vi "RTM SLSC DisableEnable.vi"(11 "Node Ptr":T1=18446744073709551615 format="%.0x") -> ()   [LabVIEW 2015, in "SLSC-12201 DIO System Explorer.lvlib"]
uses:
  SLSC-12201 DIO System Explorer.lvlib
  <vilib>/NI Veristand/Custom Device API/Custom Device Item Ref.ctl
  Shared/Constants.vi
  <vilib>/NI Veristand/Custom Device API/Custom Device API.lvlib
  Shared/SLSC-12201 DIO Shared.lvlib
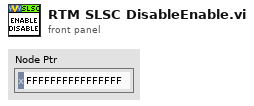
[diagram p1: front panel]
types:
  T1 = typedef "Custom Device API.lvlib/Custom Device Item Ref.ctl" = u64
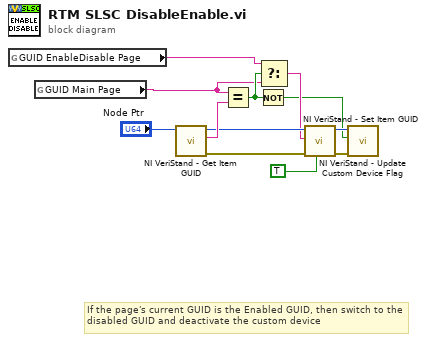
[diagram p0: block diagram]
diagram:
  # "If the page's current GUID is the Enabled GUID, then switch to the disabled GUID and deactivate the custom device"
  n1 = global read "Constants.vi" "GUID EnableDisable Page"() -> (w1:string)
  n2 = global read "Constants.vi" "GUID Main Page"() -> (w2:string)
  n3 = call <vilib>:"NI VeriStand - Get Item GUID.vi"("Item Ref in"="Node Ptr") -> ("error out"=w9:errorcluster, "GUID"=w11:string, "Item Ref out"=w6:T1)  [unwired: 8 in]
  n4 = Equal?(x=w2, y=w11) -> (x = y?=w3:bool)
  n5 = Not(x=w3) -> (.not. x?=w4:bool)
  n6 = Select(t=w1, s=w3, f=w2) -> (s? t:f=w5:string)
  n7 = call <vilib>:"NI VeriStand - Set Item GUID.vi"("Refresh System Explorer Tree? (F)"=TRUE, "error in (no error)"=w9, "GUID"=w5, "Item Ref in"=w6) -> ("error out"=w8:errorcluster, "Item Ref out"=w7:T1)  [unwired: 6 in]
  n8 = call <vilib>:"NI VeriStand - Update Custom Device Flag.vi"("error in (no error)"=w8, "Is Custom Device Active?"=w4, "Device Ref in"=w7) -> ()  [unwired: 7 in, 2 out]
